vi "Run VI Test.vi"(11 "Array":string[](array[string])) -> (2 "Message to log to console":string, 3 "exit code":i32)   [LabVIEW 2018]
doc: "This VI is a basic example used for the NI Jenkins CLI Demo"
uses:
  <vilib>/Utility/error.llb/DialogType.ctl
panel:
  in  "error IO":errorcluster
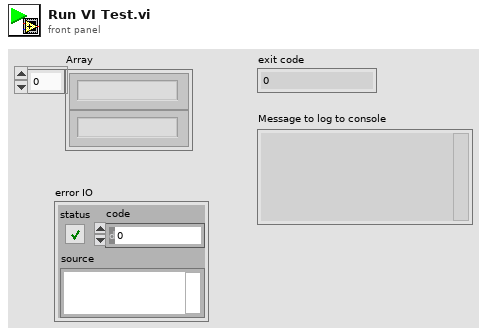
[diagram p1: front panel]
types:
  T1 = typedef "DialogType.ctl" = u16
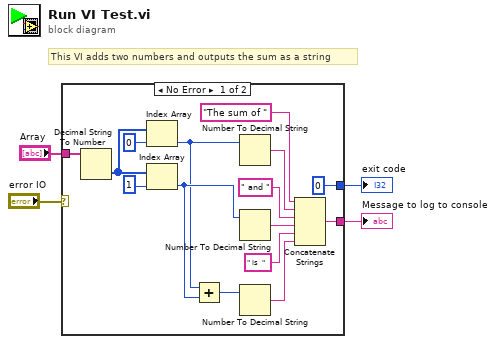
[diagram p0: block diagram]
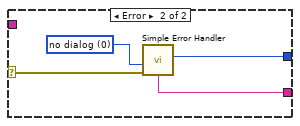
[diagram p2: hidden frame]
diagram:
  # "This VI adds two numbers and outputs the sum as a string"
  n1 = case shown="No Error" "error IO" {
    selector: "error IO" -> [_ w23]
    tunnel: [0 ("exit code") w21] -> w4
    tunnel: [w7 w20] -> w3
    tunnel: "Array" -> [w6 _]
    frame No Error {
      n2 = Decimal String To Number(string=w6) -> (number=w12:i32[])  [unwired: 2 in, 1 out]
      n3 = Index Array(array=w12, index=0) -> (element=w13:i32)
      n4 = Index Array(array=w12, index=1) -> (element=w15:i32)
      n5 = Add(x=w13, y=w15) -> (x+y=w17:i32)
      n6 = Number To Decimal String(number=w13) -> (decimal integer string=w14:string)  [unwired: 1 in]
      n7 = Number To Decimal String(number=w15) -> (decimal integer string=w16:string)  [unwired: 1 in]
      n8 = Number To Decimal String(number=w17) -> (decimal integer string=w18:string)  [unwired: 1 in]
      n9 = Concatenate Strings("The sum of " ("string"), w14, " and " ("string"), w16, " is  " ("string"), w18) -> (w7:string)
    }
    frame Error {
      w22 = T1 0 items=["no dialog", "OK message", "continue or stop message", "OK message + warnings", "continue/stop + warnings"] ("type of dialog (OK msg:1)")
      n10 = call <vilib>:"Simple Error Handler.vi"("type of dialog (OK msg:1)"=w22, "error in (no error)"=w23) -> ("code out"=w21:i32, "message"=w20:string)  [unwired: 3 in, 3 out]
    }
  }
  "exit code" <- w4
  "Message to log to console" <- w3
